vi "RT-Main-Deploy-Many.vi"(8 "error in (no error)":errorcluster, 9 "run time":u32=60, 10 "target alias":string="cRIO", 11 "configuration file path":path=path "/home/lvuser/RT_Exec_Timing.pcfg") -> (0 "error out":errorcluster)   [LabVIEW 2014]
doc: "This application launches and executes the Tag Bus Data framework configuration for the specified target alias. This is a simple example of the framework API functions, but may also be a suitable starting point for a Host UI or Thick Client that is running a local version of the framework."
uses:
  <vilib>/NI/Module Execution Interface/Engine Runtime/Engine Runtime Interface.lvclass
  <vilib>/NI/DCAF/Tag Editor Core/Framework Configuration Classes/target runtime/PL_Target Runtime.lvclass
panel:
  out "dev/nul":errorcluster
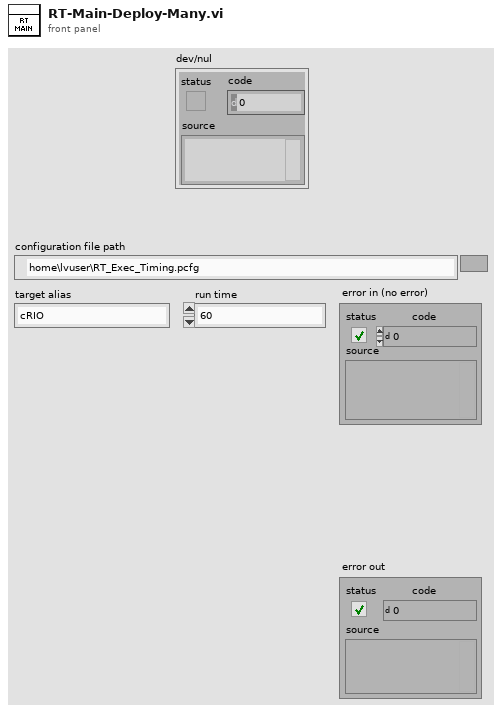
[diagram p1: front panel]
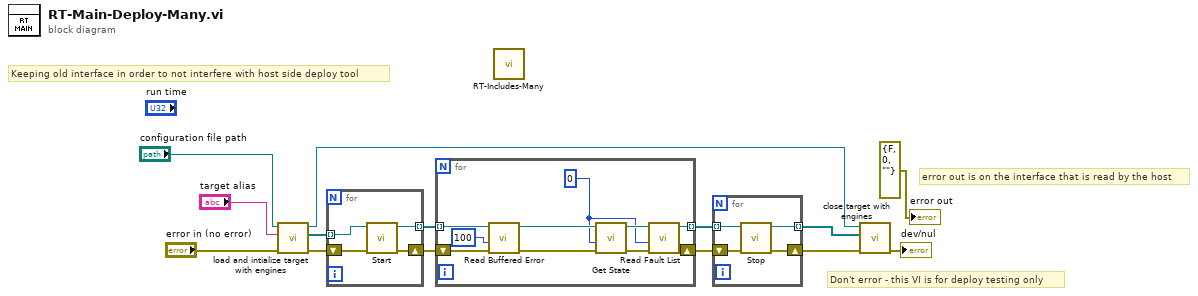
[diagram p0: block diagram]
diagram:
  # "error out is on the interface that is read by the host"
  # "Keeping old interface in order to not interfere with host side deploy tool"
  # "Don't error - this VI is for deploy testing only"
  n1 = call <vilib>:"load and intialize target with engines.vi"("error in"="error in (no error)", "target alias"="target alias", "file path"="configuration file path") -> ("error out"=w11:errorcluster, "engine runtime interfaces"=w10:refnum<class "Engine Runtime Interface.lvclass">[], "target runtime"=w8:refnum<class "PL_Target Runtime.lvclass">)  [unwired: 6 in]
  n2 = for {
    tunnel: [w18] -> w14 mode=indexing
    tunnel: w10 -> [w15] mode=indexing
    shift-right: [w17] -> w5
    shift-left: w11 -> [w16]
    n3 = call-dynamic "Start.vi"("error in"=w16, "Engine Runtime Interface in"=w15) -> ("error out"=w17:errorcluster, "Engine Runtime Interface out"=w18:refnum<class "Engine Runtime Interface.lvclass">)  [unwired: 8 in]
  }
  n4 = for {
    tunnel: w14 -> [w28] mode=indexing
    tunnel: [w21] -> w13 mode=indexing
    shift-right: [w20] -> w12
    shift-left: w5 -> [w27]
    w19 = 0 ("timeout (-1)")
    n5 = call-dynamic "Read Buffered Error.vi"("error in"=w27, "timeout in ms (0)"=100, "Engine Runtime Interface in"=w28) -> ("error out"=w25:errorcluster, "Engine Runtime Interface out"=w26:refnum<class "Engine Runtime Interface.lvclass">)  [unwired: 6 in, 1 out]
    n6 = call-dynamic "Get State.vi"("error in"=w25, "timeout (-1)"=w19, "Engine Runtime Interface in"=w26) -> ("error out"=w23:errorcluster, "Engine Runtime Interface out"=w22:refnum<class "Engine Runtime Interface.lvclass">)  [unwired: 6 in, 1 out]
    n7 = call-dynamic "Read Fault List.vi"("error in"=w23, "timeout (-1)"=w19, "Engine Runtime Interface in"=w22) -> ("error out"=w20:errorcluster, "Engine Runtime Interface out"=w21:refnum<class "Engine Runtime Interface.lvclass">)  [unwired: 6 in, 1 out]
  }
  n8 = call "RT-Includes-Many.vi"() -> ()  [unwired: 12 in]
  n9 = for {
    tunnel: w13 -> [w32] mode=indexing
    shift-right: [w29] -> w7
    shift-left: w12 -> [w31]
    tunnel: [w30] -> w2 mode=indexing
    n10 = call-dynamic "Stop.vi"("error in"=w31, "Engine Runtime Interface in"=w32) -> ("error out"=w29:errorcluster, "Engine Runtime Interface out"=w30:refnum<class "Engine Runtime Interface.lvclass">)  [unwired: 8 in]
  }
  n11 = call <vilib>:"close target with engines.vi"("error in"=w7, "Engine Runtime Interfaces"=w2, "Target Runtime"=w8) -> ("error out"=→"dev/nul":errorcluster)  [unwired: 8 in]
  "error out" <- errorcluster {"status"=FALSE, "code"=0, "source"=""} ("error out")
